vi "Display Log.vi"(11 "all rows":string[][](array[string])) -> ()   [LabVIEW 2021]
uses:
  <vilib>/Analysis/baseanly.llb/Mean (DBL).vi
  <vilib>/Analysis/NI_AALBase.lvlib
panel:
  in  "Log Data":i32(listbox)
  out "Standard Deviation of Viscosity":string
  out "Average Viscosity":string
  out "Minimum Viscosity":string
  out "Maximum Viscosity":string
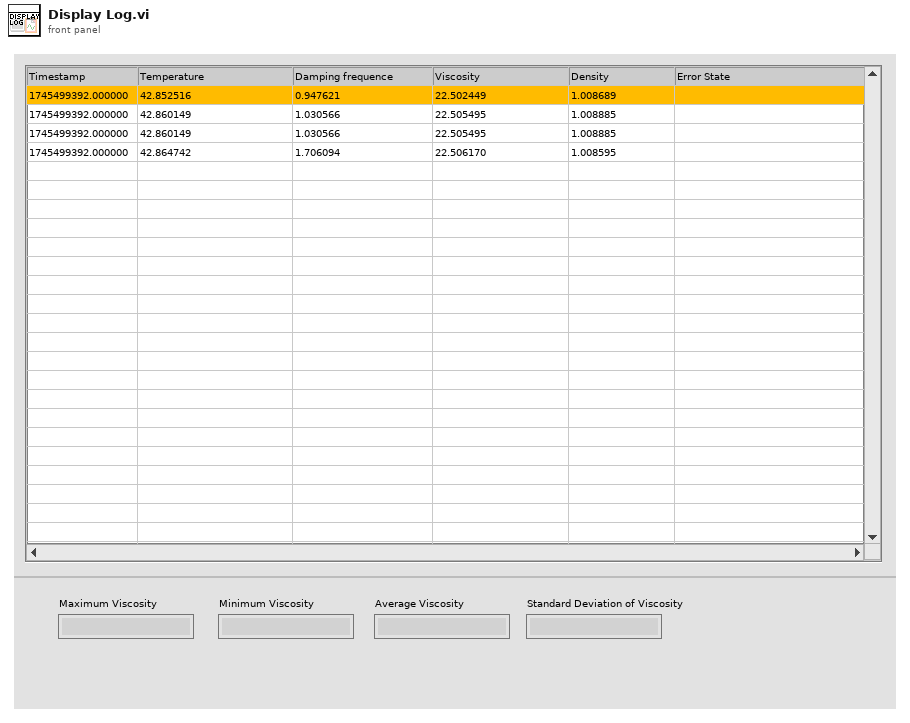
[diagram p1: front panel]
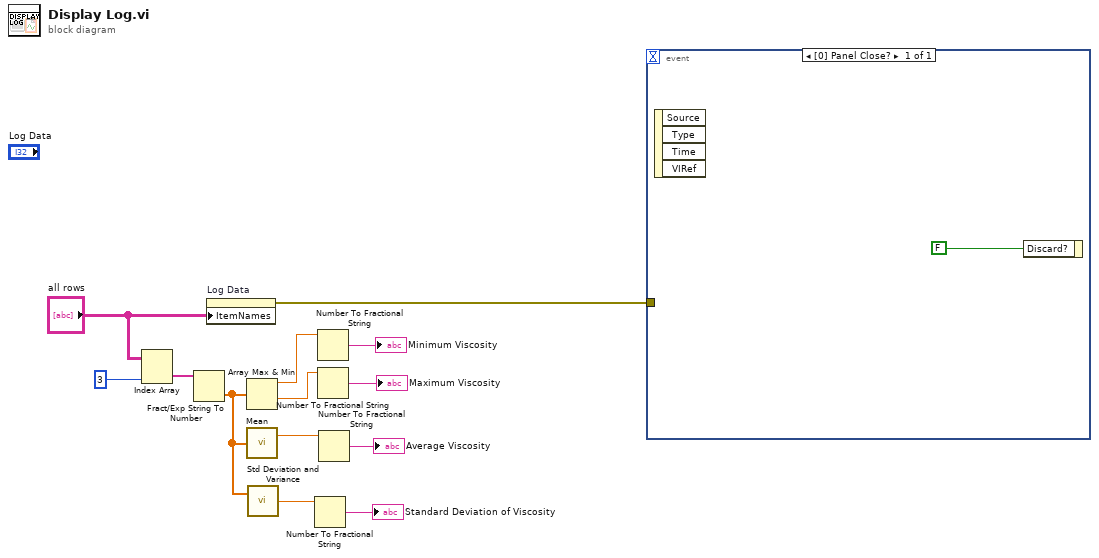
[diagram p0: block diagram]
diagram:
  n1 = Index Array(array="all rows", index (col)=3 ("disabled index (col)")) -> (element=w10:string[])  [unwired: 1 in]
  n2 = Fract/Exp String To Number(string=w10) -> (number=w3:dbl[])  [unwired: 3 in, 1 out]
  n3 = property on="Log Data" class="MCListbox (strict)"("ItemNames"="all rows") -> (error out=w13:errorcluster)  [unwired: 2 in, 1 out]
  n4 = Array Max & Min(array=w3) -> (max value=w8:dbl, min value=w7:dbl)  [unwired: 2 out]
  n5 = call-poly <vilib>:"Mean.vi"("X"=w3) -> ("mean"=w5:dbl)  [unwired: 1 out]
  n6 = call <vilib>:"Std Deviation and Variance.vi"("X"=w3) -> ("standard deviation"=w2:dbl)  [unwired: 1 in, 2 out]
  n7 = Number To Fractional String(number=w2) -> (F-format string=→"Standard Deviation of Viscosity":string)  [unwired: 3 in]
  n8 = Number To Fractional String(number=w8) -> (F-format string=→"Minimum Viscosity":string)  [unwired: 3 in]
  n9 = Number To Fractional String(number=w7) -> (F-format string=→"Maximum Viscosity":string)  [unwired: 3 in]
  n10 = Number To Fractional String(number=w5) -> (F-format string=→"Average Viscosity":string)  [unwired: 3 in]
  n11 = event shown="[0] Panel Close?" {
    selector: _ -> [_]
    dyn-events: _ -> [_]
    timeout: _ -> [_]
    tunnel: w13 -> [_]
    event Panel Close? {
      n12 = event-data() -> ()  [unwired: 1 in, 4 out]
      n13 = event-data("Discard?"=FALSE) -> ()  [unwired: 1 in, 1 out]
    }
  }
